vi "Index Point Cal Eval.vi"(8 "error in (no error)":errorcluster caption="错误输入（无错误）", 9 "kOffsInit":i32, 10 "AsicSignal":dbl, 11 "asicHandle":i32) -> (0 "error out":errorcluster caption="错误输出", 1 "kOffsInit out":i32, 3 "function return":i32)   [LabVIEW 2018]
doc: "extern int __stdcall APSxIndexPointCalEval (int asicHandle, IN double AsicSignal, OUT int * kOffsInit);"
uses:
  APSx.dll/APSx.dll
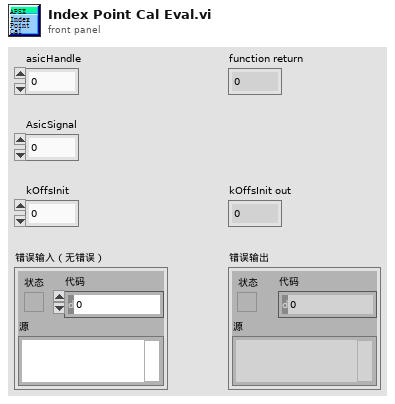
[diagram p1: front panel]
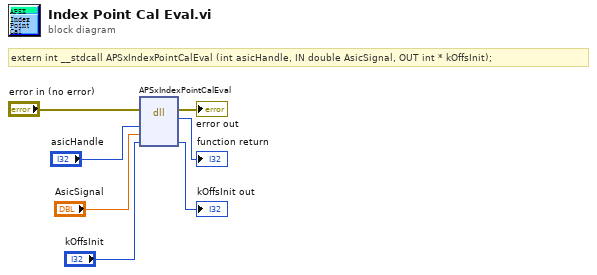
[diagram p0: block diagram]
diagram:
  # "extern int __stdcall APSxIndexPointCalEval (int asicHandle, IN double AsicSignal, OUT int * kOffsInit);"
  n1 = dll-call lib="PTH2[abs D项目Feng恒隆项目Labview传感器对中台SourcesAPSx.dllAPSx.*" fn="APSxIndexPointCalEval"(error in="error in (no error)", "asicHandle"="asicHandle", "AsicSignal"="AsicSignal", "kOffsInit"="kOffsInit") -> (error out=→"error out":errorcluster, →"function return":i32, "kOffsInit"=→"kOffsInit out":i32)  [unwired: 4 in, 1 out]
